vi "Solve PnP (P3P).vi"(6 "Camera Parameters":T7, 8 "error in (no error)":errorcluster, 11 "Point Correspondence Set":T1) -> (0 "error out":errorcluster, 3 "Pose":T4)   [LabVIEW 2020, in "g_ar_toolkit.ar.lvlib"]
uses:
  g_ar_toolkit.ar.lvlib
  g_ar_toolkit.common/Camera Parameters.ctl
  g_ar_toolkit.common/Camera Matrix.ctl
  g_ar_toolkit.common/Camera Distortion Coefficients.ctl
  Pose.ctl
  rvec.ctl
  g_ar_toolkit.common/tvec.ctl
  Point Correspondence Set.ctl
  g_ar_toolkit.common/Object Point (Float).ctl
  g_ar_toolkit.common/Image Point (Float).ctl
  SolvePnPFlags.ctl
  g_ar_toolkit.common/Module Path.vi
  <vilib>/Utility/error.llb/Error Cluster From Error Code.vi
  g_ar_toolkit.common/g_ar_toolkit.common.lvlib
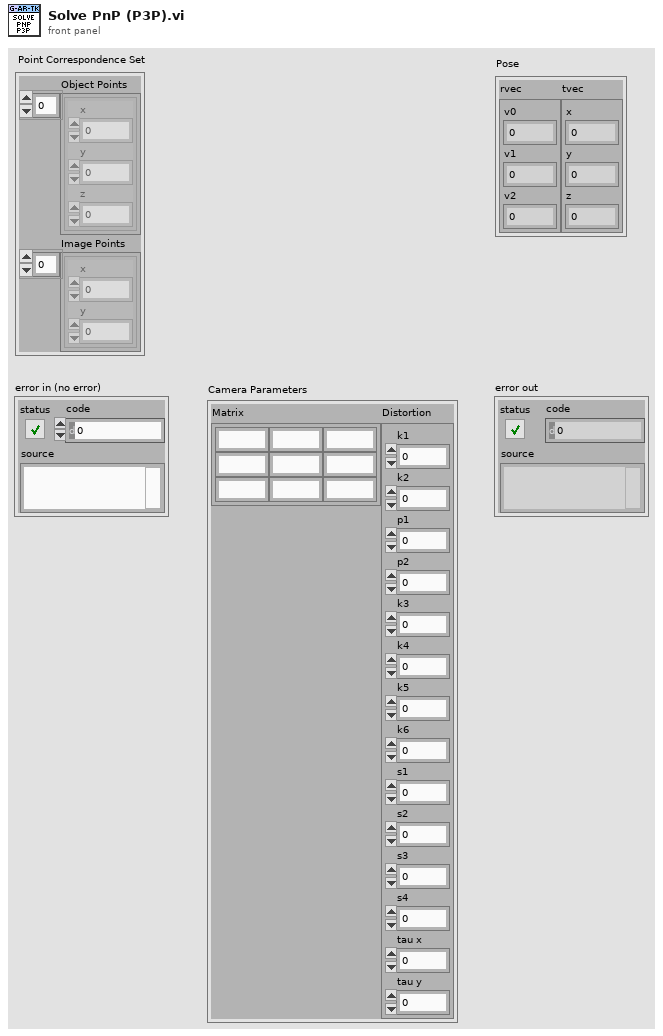
[diagram p1: front panel]
types:
  T1 = typedef "g_ar_toolkit.ar.lvlib/Point Correspondence Set.ctl" = cluster{"Object Points":T2[], "Image Points":T3[]}
  T2 = typedef "g_ar_toolkit.common.lvlib/Object Point (Float).ctl" = cluster{"x":dbl, "y":dbl, "z":dbl}
  T3 = typedef "g_ar_toolkit.common.lvlib/Image Point (Float).ctl" = cluster{"x":dbl, "y":dbl}
  T4 = typedef "g_ar_toolkit.ar.lvlib/Pose.ctl" = cluster{"rvec":T5, "tvec":T6}
  T5 = typedef "g_ar_toolkit.ar.lvlib/rvec.ctl" = cluster{"v0":dbl, "v1":dbl, "v2":dbl}
  T6 = typedef "g_ar_toolkit.ar.lvlib/tvec.ctl" = cluster{"x":dbl, "y":dbl, "z":dbl}
  T7 = typedef "g_ar_toolkit.common.lvlib/Camera Parameters.ctl" = cluster{"Matrix":T8, "Distortion":T9}
  T8 = typedef "g_ar_toolkit.common.lvlib/Camera Matrix.ctl" = cluster{"m 0,0":dbl, "m 0,1":dbl, "m 0,2":dbl, "m 1,0":dbl, "m 1,1":dbl, "m 1,2":dbl, "m 2,0":dbl, "m 2,1":dbl, "m 2,2":dbl}
  T9 = typedef "g_ar_toolkit.common.lvlib/Camera Distortion Coefficients.ctl" = cluster{"k1":dbl, "k2":dbl, "p1":dbl, "p2":dbl, "k3":dbl, "k4":dbl, "k5":dbl, "k6":dbl, "s1":dbl, "s2":dbl, "s3":dbl, "s4":dbl, "tau x":dbl, "tau y":dbl}
  T10 = typedef "g_ar_toolkit.ar.lvlib/SolvePnPFlags.ctl" = enum8{"SOLVEPNP_ITERATIVE", "SOLVEPNP_EPNP", "SOLVEPNP_P3P", "SOLVEPNP_AP3P", "SOLVEPNP_IPPE", "SOLVEPNP_IPPE_SQUARE", "SOLVEPNP_SQPNP"}
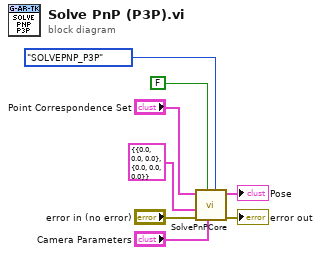
[diagram p0: block diagram]
diagram:
  n1 = call "SolvePnPCore.vi"("Solve PnP Flags"=SolvePnPFlags."SOLVEPNP_P3P", "Camera Parameters"="Camera Parameters", "Use Pose Guess"=FALSE ("Use Iterative"), "error in (no error)"="error in (no error)", "Pose (Estimate) in"=T4 {"rvec"={"v0"=0.0, "v1"=0.0, "v2"=0.0}, "tvec"={"x"=0.0, "y"=0.0, "z"=0.0}} ("Pose (Estimate)"), "Point Correspondence Set"="Point Correspondence Set") -> ("error out"=→"error out":errorcluster, "Pose"=→"Pose":T4)  [unwired: 4 in]
